vi "Set Value.vi"(8 "error in (no error)":errorcluster, 10 "Value":string, 11 "Option in":refnum<class "Option.lvclass">) -> (0 "error out":errorcluster, 3 "Option out":refnum<class "Option.lvclass">)   [LabVIEW 2011, in "Option Parser.lvlib" / "Option.lvclass"]
doc: "Sets the value of the option.\n\nIf it is just a flag the value is ignored but it is then considered set."
uses:
  Option.lvclass
  Option.lvclass/Option.ctl
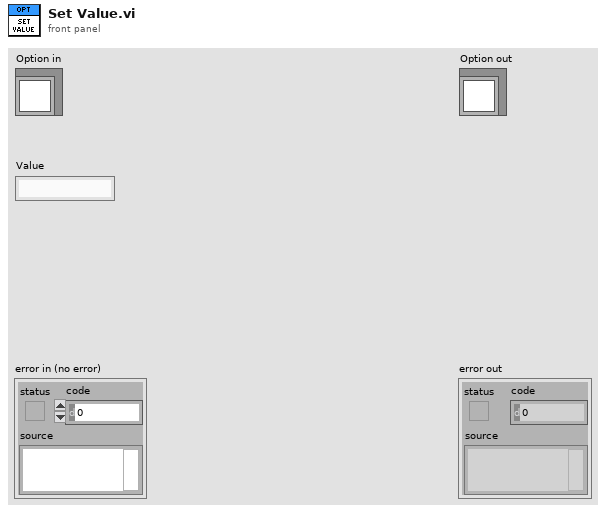
[diagram p1: front panel]
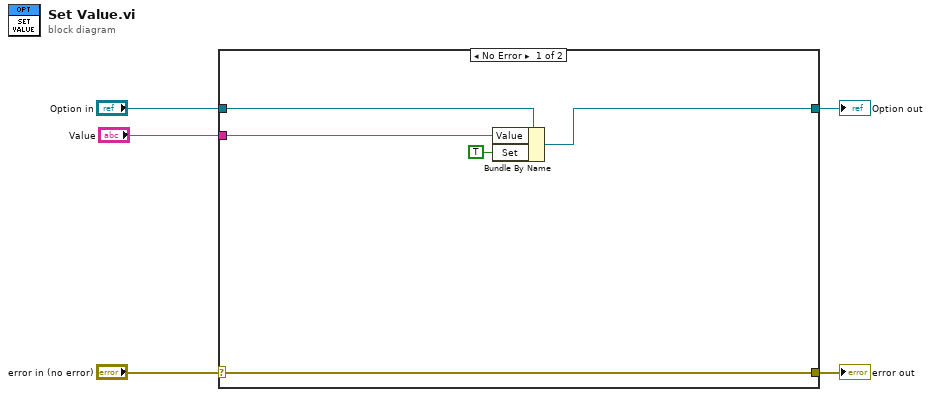
[diagram p0: block diagram]
diagram:
  n1 = case shown="No Error" "error in (no error)" {
    selector: "error in (no error)" -> [w9 w12]
    tunnel: [w9 w12] -> w4
    tunnel: [w8 w11] -> w2
    tunnel: "Option in" -> [w10 w11]
    tunnel: "Value" -> [w7 _]
    frame No Error {
      n2 = Bundle By Name(cluster=w10, "Value"=w7, "Set"=TRUE) -> (w8:refnum<class "Option.lvclass">)
    }
    frame Error {
    }
  }
  "error out" <- w4
  "Option out" <- w2
